vi "Send Data to Core.vi"(8 "error in (no error)":errorcluster, 10 "Data":string, 11 "WS Test Client in":refnum<class "WS Test Client.lvclass">) -> (0 "error out":errorcluster, 3 "WS Test Client out":refnum<class "WS Test Client.lvclass">)   [LabVIEW 2021, in "Echo Broadcast Test Without Server Manager.lvlib" / "WS Test Client.lvclass"]
uses:
  WS Test Client.lvclass
  WS Test Client.lvclass/WS Test Client.ctl
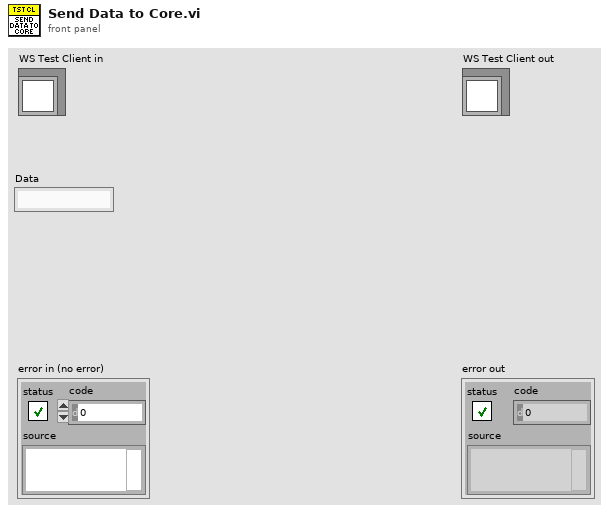
[diagram p1: front panel]
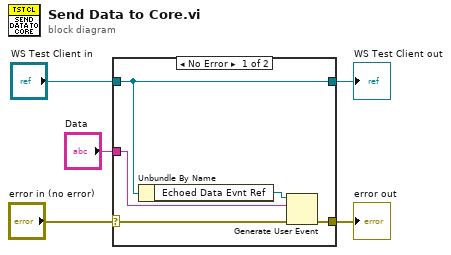
[diagram p0: block diagram]
diagram:
  n1 = case shown="No Error" "error in (no error)" {
    selector: "error in (no error)" -> [w8 w12]
    tunnel: [w7 w12] -> w4
    tunnel: [w10 w11] -> w2
    tunnel: "WS Test Client in" -> [w10 w11]
    tunnel: "Data" -> [w6 _]
    frame No Error {
      n2 = Unbundle By Name(w10) -> ("Echoed Data Evnt Ref"=w9:refnum<user-event>)
      n3 = Generate User Event(user event=w9, event data cluster=w6, error in=w8) -> (error out=w7:errorcluster)  [unwired: 1 in, 1 out]
    }
    frame Error {
    }
  }
  "error out" <- w4
  "WS Test Client out" <- w2
